vi "Generate Session Management Client.vi"(8 "error in (no error)":errorcluster) -> (0 "error out":errorcluster)   [LabVIEW 2020, in "MeasurementLink Proto Builds.lvlib"]
uses:
  MeasurementLink Proto Builds.lvlib
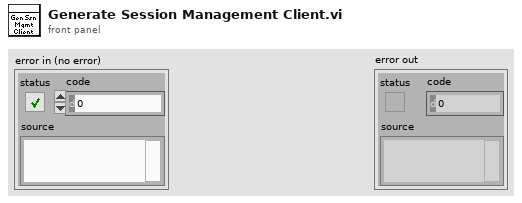
[diagram p1: front panel]
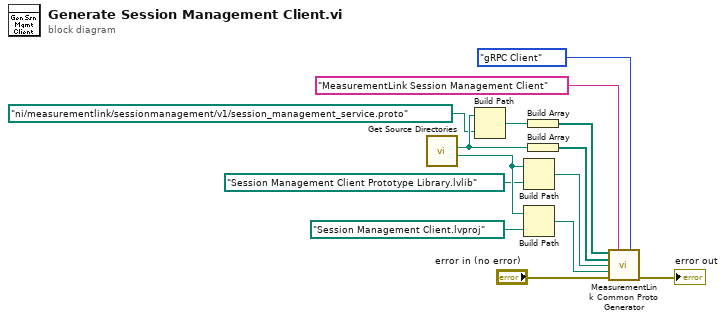
[diagram p0: block diagram]
diagram:
  n1 = call "Get Source Directories.vi"() -> ("Runtime Dir"=w9:path, "Protos Dir"=w5:path)  [unwired: 9 in, 1 out]
  n2 = Build Path(base path=w5, name or relative path=path "ni/measurementlink/sessionmanagement/v1/session_management_service.proto" ("Proto File Path")) -> (appended path=w6:path)
  n3 = Build Path(base path=w9, name or relative path=path "Session Management Client Prototype Library.lvlib") -> (appended path=w7:path)
  n4 = Build Path(base path=w9, name or relative path=path "Session Management Client.lvproj" ("Target Project")) -> (appended path=w10:path)
  n5 = Build Array(w6) -> (w12:path[])
  n6 = Build Array(w5) -> (w13:path[])
  n7 = call "MeasurementLink Common Proto Generator.vi"("Proto File Path"=w12, "Generated Library Full Name"="MeasurementLink Session Management Client" ("Generated Library Name"), "Generate"=enum16{"gRPC Server", "gRPC Client", "Both"}."gRPC Client", "Import Paths"=w13, "Prototype Library"=w7, "Target Project"=w10, "error in (no error)"="error in (no error)") -> ("error out"=→"error out":errorcluster)  [unwired: 8 in]
